vi "DIMPowerSupply.destructor.vi"(0 "i ref in":refnum<vi>, 5 "error in (no error)":errorcluster) -> (19 "error out":errorcluster)   [LabVIEW 2014, in "DIMPowerSupply.lvlib"]
doc: "This is the destructor of a class.\n\nLicense Agreement for this software:\n\nCopyright (C)\nGesellschaft für Schwerionenforschung, GSI\nPlanckstr. 1\n64291 Darmstadt\nGermany\n\nContact: D.Beck@gsi.de \n\nThis program is free software; you can redistribute it and/or modify it under the terms of the \nGNU General Public License as published by the Free Software Foundation; either version 2 of \nthe license, or (at your option) any later version.\n\nThis program is distributed in the hope that it will be useful, but WITHOUT ANY WARRANTY; \nwithout even the implied warranty of MERCHANTABILITY or FITNESS FOR A PARTICULAR PURPOSE. See the GNU General License for more details (http://www.gnu.org).\n\nGesellschaft für Schwerionenforschung, GSI\nPlanckstr. 1, 64291 Darmstadt, Germany\nFor all questions and ideas contact: M.Richter@gsi.de, H.Brand@gsi.de or D.Beck@gsi.de.\nLast update: 16-JUN-2004"
uses:
  DIMPowerSupply.lvlib
  CSCore/CSApplicationBaseClasses/PSChannelBase/PSChannelBase.lvlib
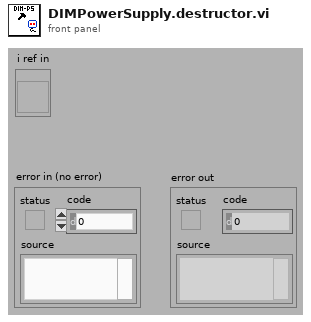
[diagram p1: front panel]
types:
  T1 = enum16{"SetAttribute", "GetAttribute", "CreateAttribute", "DestroyAttribute", "DestroyAllAtributes"}
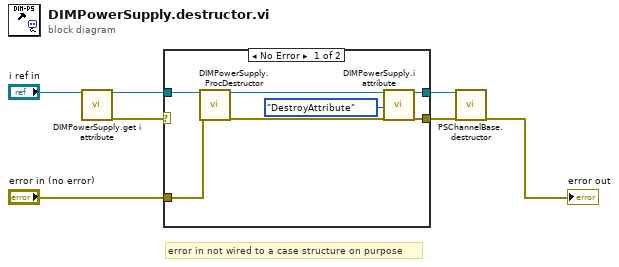
[diagram p0: block diagram]
diagram:
  # "error in not wired to a case structure on purpose"
  n1 = call "DIMPowerSupply.get i attribute.vi"("i ref in"="i ref in") -> ("i ref out"=w2:refnum<vi>, "error out"=w1:errorcluster)  [unwired: 16 in, 1 out]
  n2 = case shown="No Error" w1 {
    tunnel: [w13 w16] -> w7
    tunnel: [w12 w15] -> w6
    tunnel: "error in (no error)" -> [w9 w15]
    tunnel: w2 -> [w8 w16]
    frame No Error {
      n3 = call "DIMPowerSupply.ProcDestructor.vi"("i ref in"=w8, "error in (no error)"=w9) -> ("i ref out"=w11:refnum<vi>, "error out"=w10:errorcluster)  [unwired: 16 in]
      n4 = call "DIMPowerSupply.i attribute.vi"("VI Refnum"=w11, "Action"=T1."DestroyAttribute", "error in (no error)"=w10) -> ("VI Refnum out"=w13:refnum<vi>, "error out"=w12:errorcluster)  [unwired: 14 in, 1 out]
    }
    frame Error {
    }
  }
  n5 = call "PSChannelBase.destructor.vi"("i ref in"=w7, "error in (no error)"=w6) -> ("error out"=→"error out":errorcluster)  [unwired: 17 in]
